vi "CW - Main.vi"() -> ()   [LabVIEW 2017]
doc: "Car Wash Automaion Application VI"
uses:
  Controls/CW - Wash Options.ctl
  Controls/CW - Car Position Control.ctl
  Controls/CW - Car Wash Indicators.ctl
  Controls/CW - Car Wash SM States.ctl
  Controls/CW -  Master Cluster.ctl
panel:
  in  "current time":timestamp
  in  "Stop":bool
  out "Elapsed Time (sec)":dbl format="%#.2g"
  out "Wash Indicators":T1
  in  "Car Position Slider":T2 scale=0.0..4.0
  out "Wash Entry":bool
  in  "Start":bool
  in  "Wash Options":T3
  # "Entry Console"
  # "Car Wash Display"
  # "The wash options controls allow you to determine which cycles will be performed.  \n\nIf none are selected, the High Pressure Wash cycle is the default.  \n\nOnce the start button is clicked, the wash begins."
  # "The Wash Entry LED indicates whether or not the wash in vacant or in use.\n\nThe Wash Indicator LEDs indicate the current status when the wash is in use.\n\nThe Elapsed Time indicator shows the progress for the current cycle, only if it is a timed cycle."
  # "Car Position Simulation"
  # "The Car Position Slider allows you to simulate the position of a vehicle in the wash.\n\nThe vehicle must be at the correct station for the each wash cycle to work.  The cycles that are completed at each station are indicated below the station number.\n\nIf the Vehicle Out of Position LED above is green, adjust your position to the appropraite station."
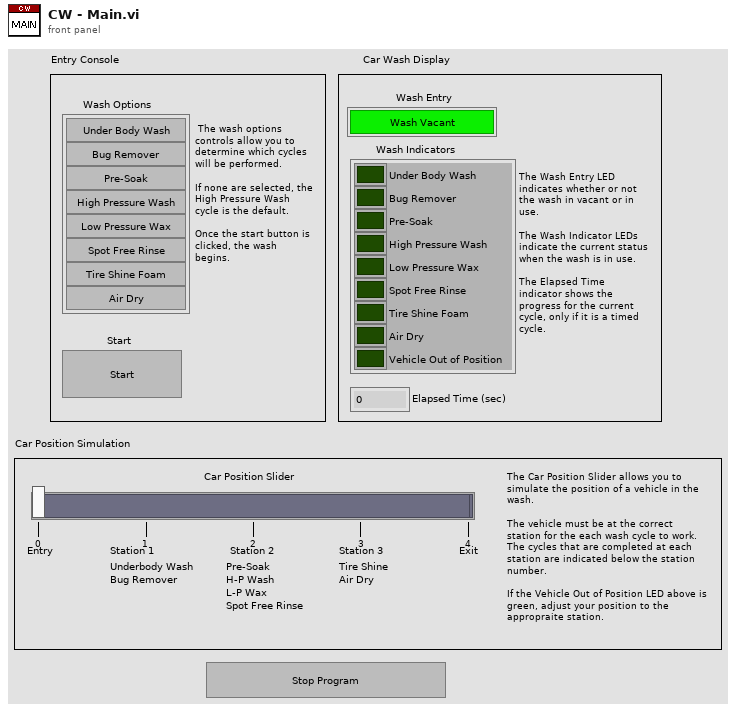
[diagram p1: front panel]
types:
  T1 = typedef "CW - Car Wash Indicators.ctl" = cluster{"Under Body Wash":bool, "Bug Remover":bool, "Pre-Soak":bool, "High Pressure Wash":bool, "Low Pressure Wax":bool, "Spot Free Rinse":bool, "Tire Shine Foam":bool, "Air Dry":bool, "Vehicle Out of Position":bool}
  T2 = typedef "CW - Car Position Control.ctl" = i32
  T3 = typedef "CW - Wash Options.ctl" = cluster{"Under Body Wash":bool, "Bug Remover":bool, "Pre-Soak":bool, "High Pressure Wash":bool, "Low Pressure Wax":bool, "Spot Free Rinse":bool, "Tire Shine Foam":bool, "Air Dry":bool}
  T4 = typedef "CW -  Master Cluster.ctl" = cluster{"Expected_position":i32, "Current_position":i32, "Elapsed Time (sec)":dbl, "Start Timer":bool, "Wash Entry":bool, "Controls Enable":bool, "Time Elapsed":bool, "Wash Step done":bool, "Wash Options":T3, "Wash Indicators":T1}
  T5 = typedef "CW - Car Wash SM States.ctl" = enum16{"Initialize", "Poll", "WaitTime at CW", "Get Data", "Unable/Disable Controls", "Update Indicators", "Start CW", "Entry", "Station 1", "Station 2", "Station 3", "Exit CarWash", "Exit", "Error"}
  T6 = cluster{"Wash Indicators[0]":bool, "Wash Indicators[1]":bool, "Wash Indicators[2]":bool, "Wash Indicators[3]":bool, "Wash Indicators[4]":bool, "Wash Indicators[5]":bool, "Wash Indicators[6]":bool, "Wash Indicators[7]":bool, "Wash Indicators[8]":bool}
  T7 = enum8{"Enabled", "Disabled", "Disabled and Grayed Out"}
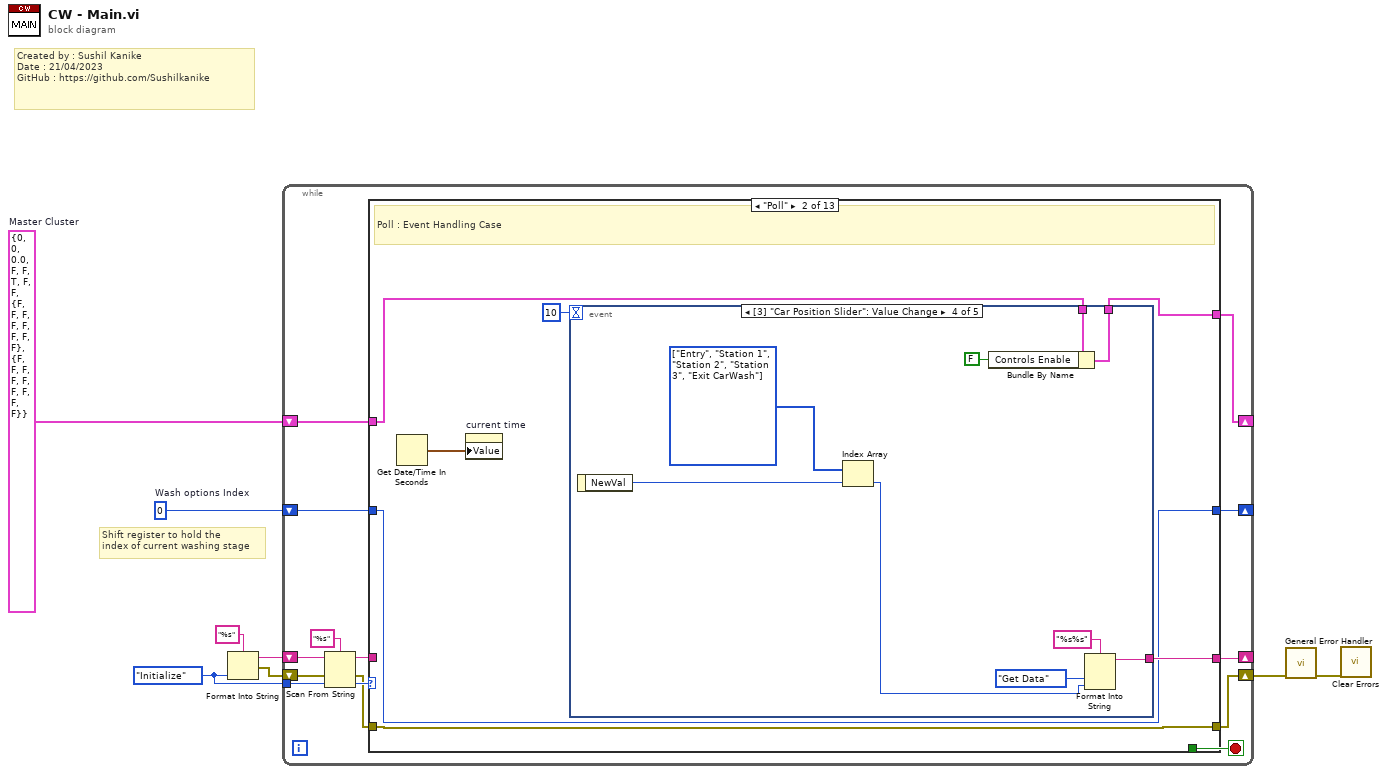
[diagram p0: block diagram]
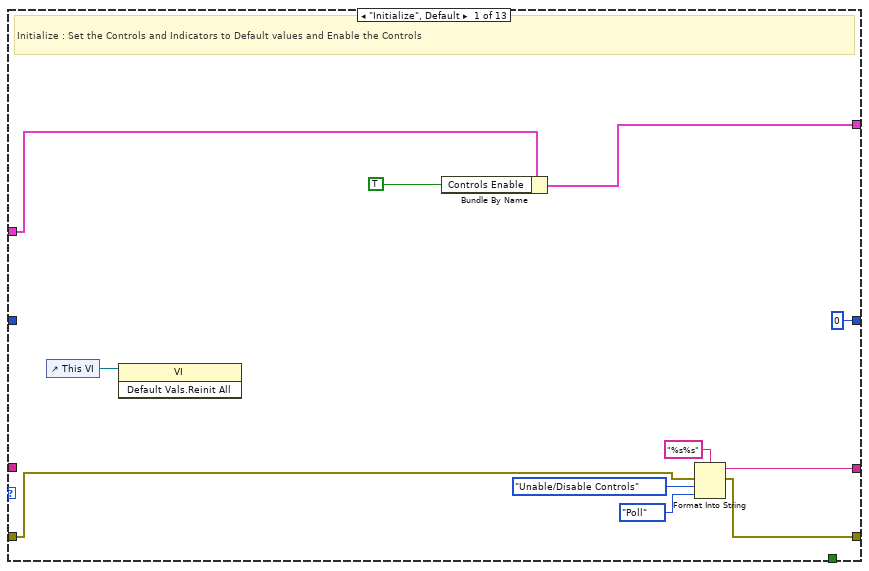
[diagram p2: hidden frame]
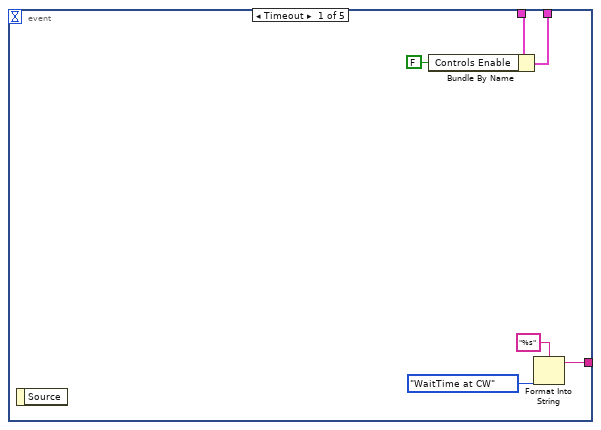
[diagram p3: hidden frame]
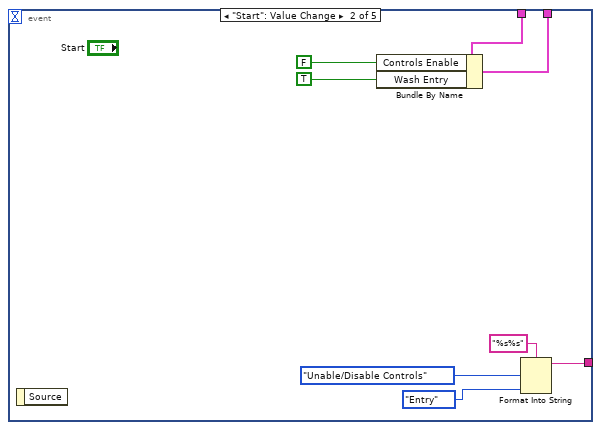
[diagram p4: hidden frame]
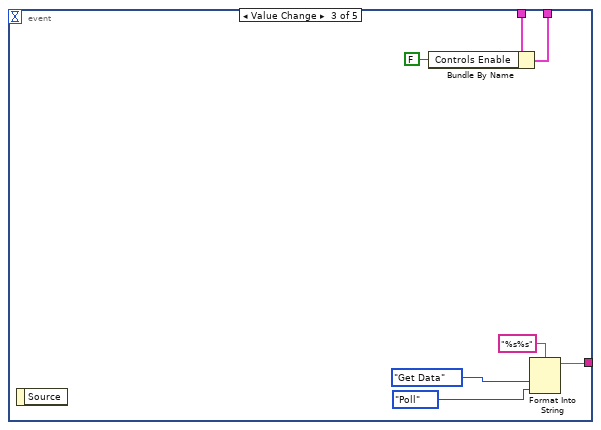
[diagram p5: hidden frame]
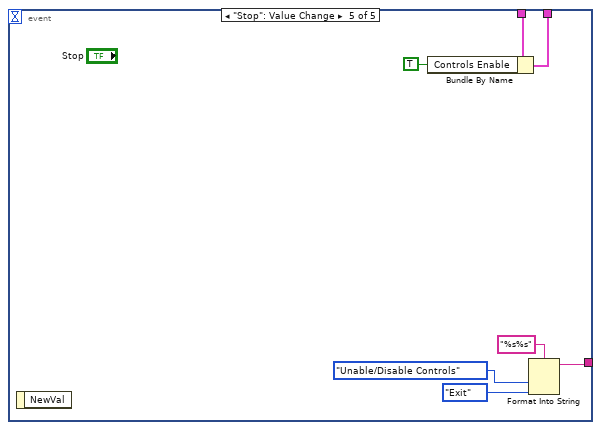
[diagram p6: hidden frame]
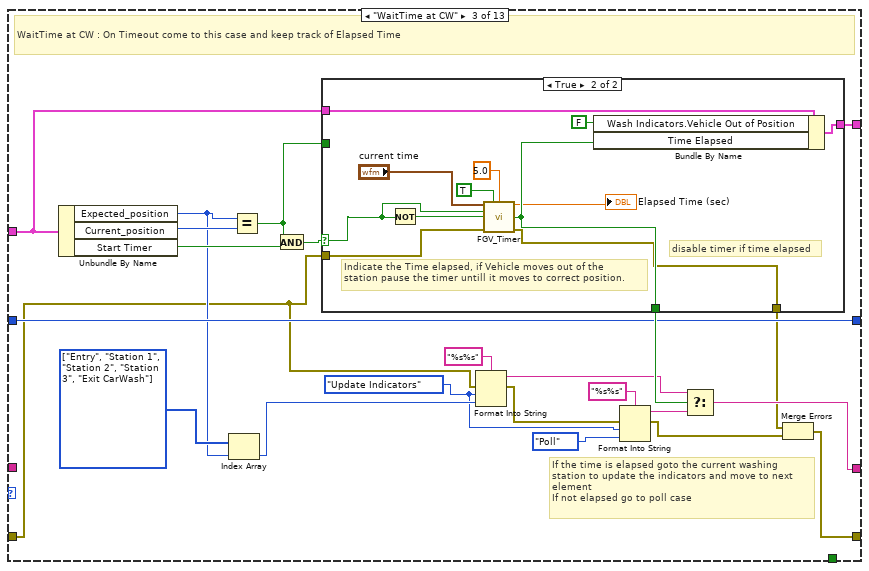
[diagram p7: hidden frame]
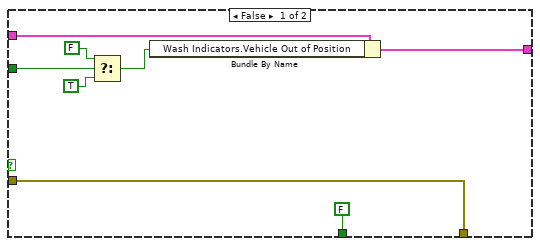
[diagram p8: hidden frame]
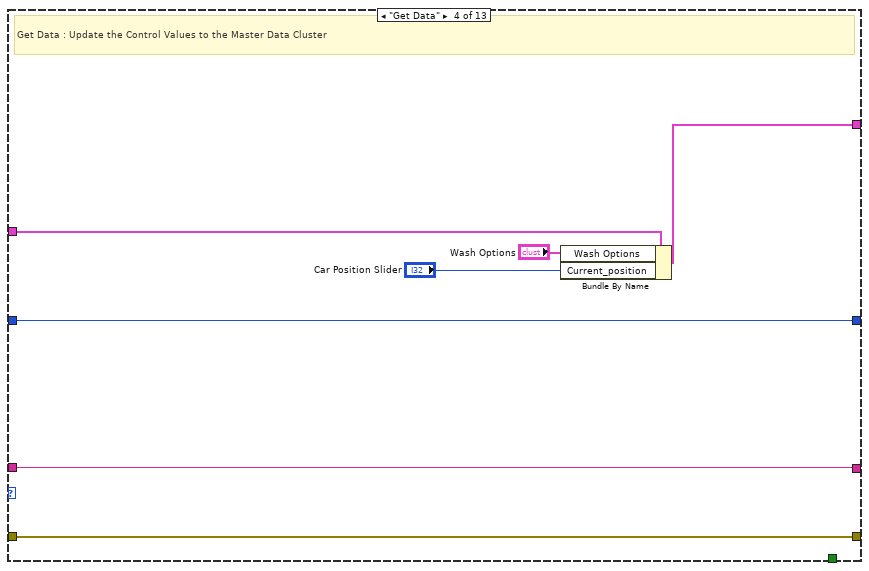
[diagram p9: hidden frame]
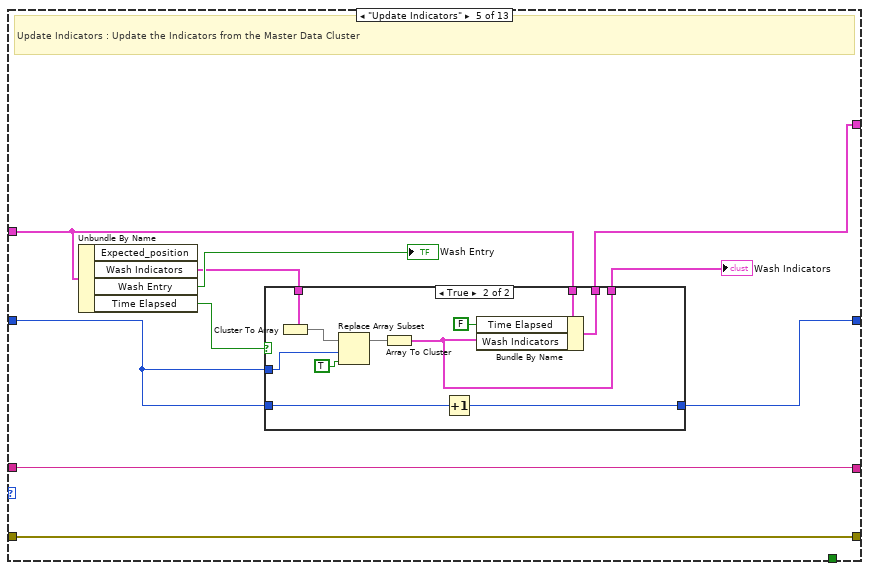
[diagram p10: hidden frame]
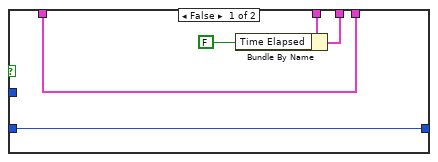
[diagram p11: hidden frame]
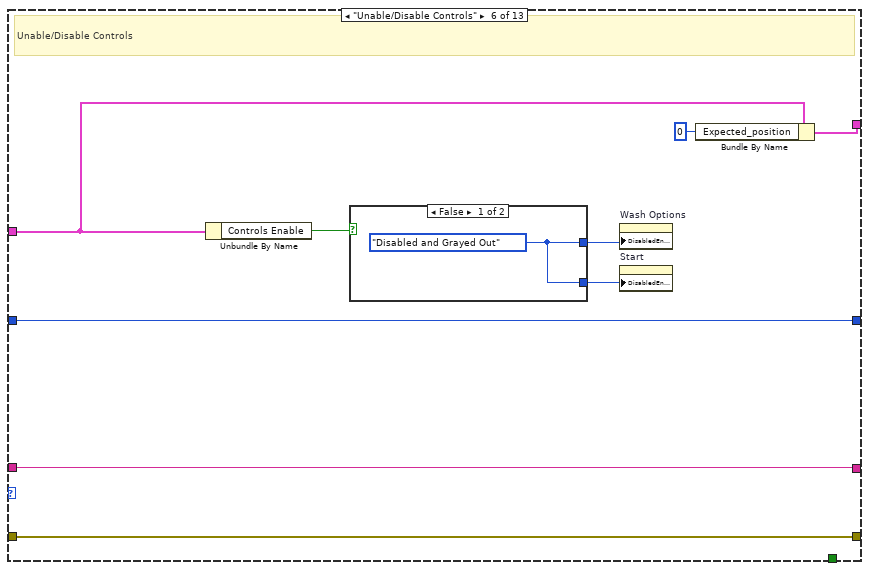
[diagram p12: hidden frame]
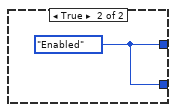
[diagram p13: hidden frame]
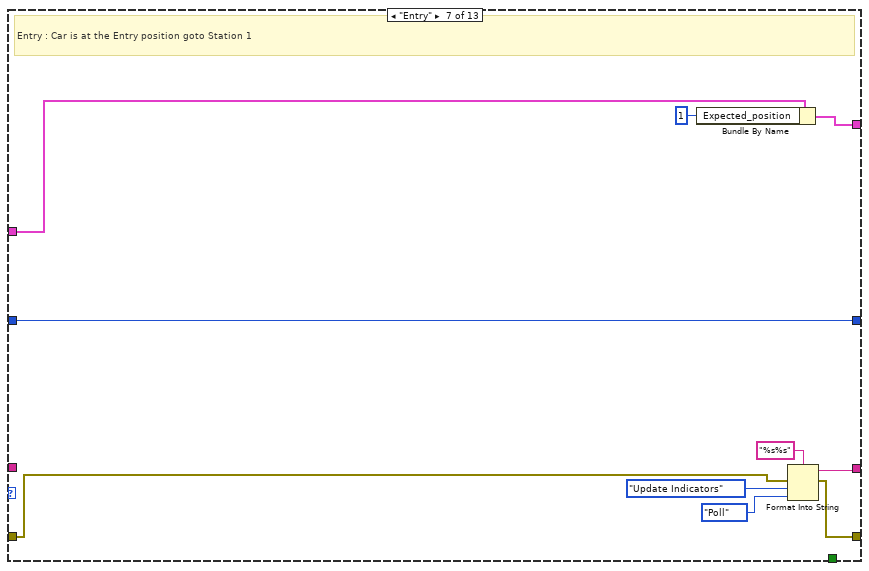
[diagram p14: hidden frame]
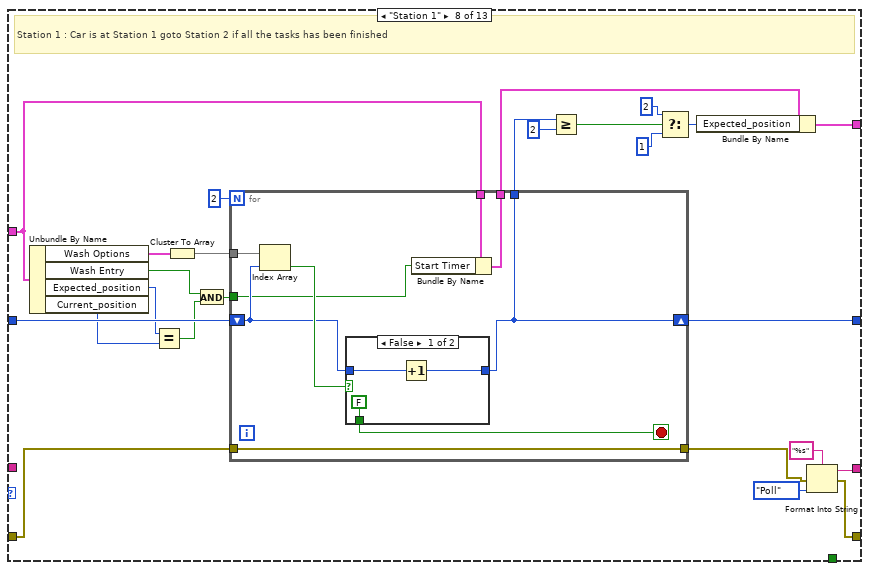
[diagram p15: hidden frame]
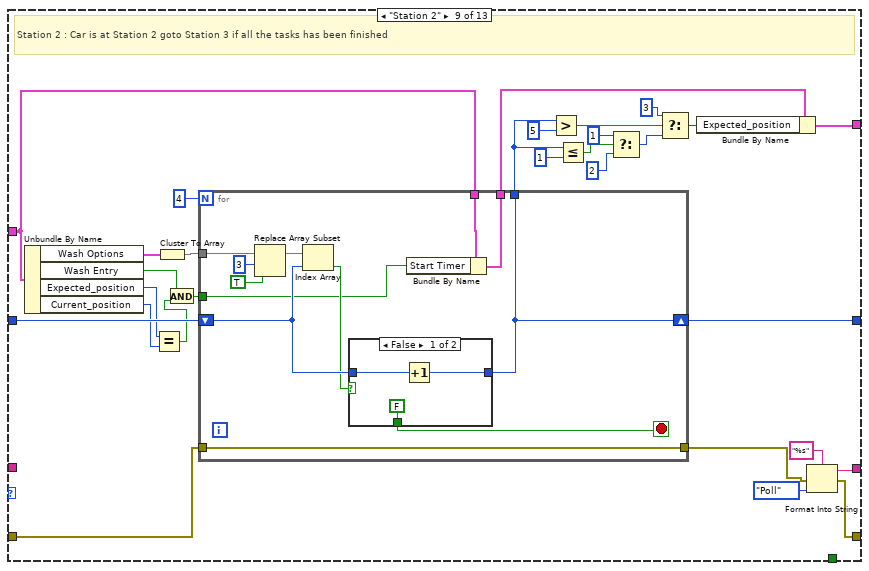
[diagram p17: hidden frame]
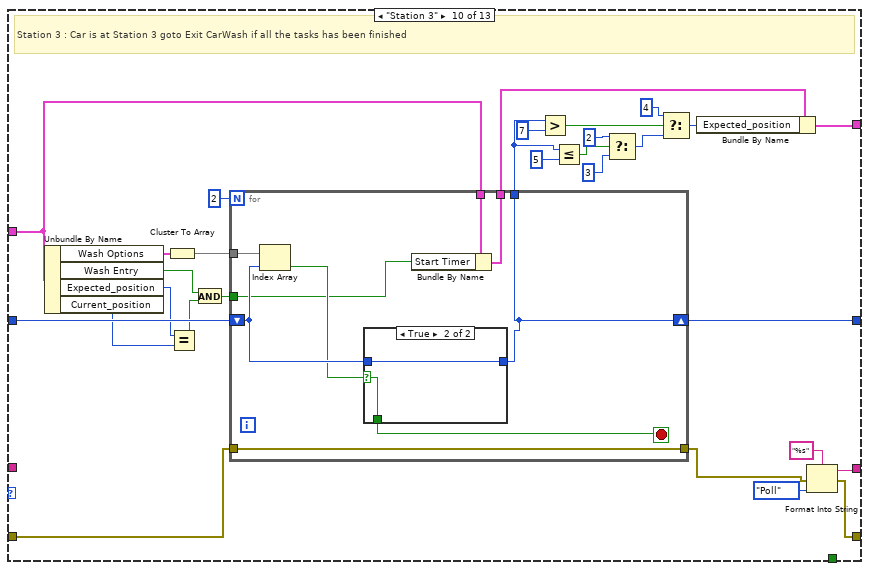
[diagram p19: hidden frame]
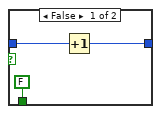
[diagram p20: hidden frame]
diagram:
  w4 = 0  # Wash options Index
  w5 = T4 {"Expected_position"=0, "Current_position"=0, "Elapsed Time (sec)"=0.0, "Start Timer"=FALSE, "Wash Entry"=FALSE, "Controls Enable"=TRUE, "Time Elapsed"=FALSE, "Wash Step done"=FALSE, "Wash Options"={"Under Body Wash"=FALSE, "Bug Remover"=FALSE, "Pre-Soak"=FALSE, "High Pressure Wash"=FALSE, "Low Pressure Wax"=FALSE, "Spot Free Rinse"=FALSE, "Tire Shine Foam"=FALSE, "Air Dry"=FALSE}, "Wash Indicators"={"Under Body Wash"=FALSE, "Bug Remover"=FALSE, "Pre-Soak"=FALSE, "High Pressure Wash"=FALSE, "Low Pressure Wax"=FALSE, "Spot Free Rinse"=FALSE, "Tire Shine Foam"=FALSE, "Air Dry"=FALSE, "Vehicle Out of Position"=FALSE}}  # Master Cluster
  w6 = CW_-_Car_Wash_SM_States."Initialize" ("Car Wash SM States")
  # "Created by : Sushil Kanike\nDate : 21/04/2023 \nGitHub : https://github.com/Sushilkanike"
  # "Shift register to hold the\nindex of current washing stage"
  n1 = Format Into String(format string="%s", w6) -> (resulting string=w7:string, error out=w8:errorcluster)  [unwired: 2 in]
  n2 = while {
    shift-right: [w17] -> _
    shift-left: w7 -> [w16]
    tunnel: w6 -> [w21]
    shift-right: [w14] -> _
    shift-left: w5 -> [w15]
    shift-right: [w13] -> _
    shift-left: w4 -> [w11]
    shift-right: [w9] -> w2
    shift-left: w8 -> [w22]
    stop <- w18 stop-if-true
    n3 = Scan From String(format string="%s", input string=w16, error in=w22, default 1=w21) -> (remaining string=w12:string, error out=w10:errorcluster, output 1=w20:T5)  [unwired: 1 in, 1 out]
    n4 = case shown="\"Poll\"" w20 {
      tunnel: [_ _ _ _ _ _ _ _ _ _ _ TRUE _] -> w18
      tunnel: [w33 w39 w94 w122 w136 w155 w170 w197 w239 w285 w319 w327 w333] -> w17
      tunnel: w15 -> [w28 w37 w93 w127 w129 w159 w173 w193 w222 w281 w324 w329 w335]
      tunnel: [w27 w36 w92 w126 w133 w158 w174 w184 w242 w288 w325 w329 w335] -> w14
      tunnel: w11 -> [_ w38 w89 w123 w131 w156 w169 w192 w234 w279 w305 w328 w334]
      tunnel: [0 w38 w89 w123 w130 w156 w169 w191 w229 w274 w305 w328 w334] -> w13
      tunnel: w12 -> [_ _ _ w122 w136 w155 _ _ _ _ _ w327 w333]
      tunnel: w10 -> [w24 w34 w82 w121 w128 w154 w166 w177 w216 w262 w304 w326 w332]
      tunnel: [w23 w34 w78 w121 w128 w154 w165 w176 w214 w260 w303 w326 w332] -> w9
      frame "Initialize", Default {
        # "Initialize : Set the Controls and Indicators to Default values and Enable the Controls"
        n5 = control-ref of="This VI"() -> (w30:refnum<vi>)
        n6 = invoke class="VI" method="Default Vals.Reinit All"(reference=w30) -> ()  [unwired: 2 in, 3 out]
        n7 = Bundle By Name(cluster=w28, "Controls Enable"=TRUE) -> (w27:T4)
        n8 = Format Into String(format string="%s%s", error in=w24, CW_-_Car_Wash_SM_States."Unable/Disable Controls" ("Car Wash SM States"), CW_-_Car_Wash_SM_States."Poll" ("Car Wash SM States")) -> (resulting string=w33:string, error out=w23:errorcluster)  [unwired: 1 in]
      }
      frame "Poll" {
        # "Poll : Event Handling Case"
        n9 = Get Date/Time In Seconds() -> (seconds since 1Jan1904=w35:timestamp)
        n10 = property on="current time" class="AbsTime (strict)"("Value"=w35) -> ()  [unwired: 2 in, 2 out]
        n11 = event shown="[3] \"Car Position Slider\": Value Change" {
          selector: _ -> [_ _ _ _ _]
          dyn-events: _ -> [_ _ _ _ _]
          timeout: 10 -> [_ _ _ _ _]
          tunnel: [w46 w52 w59 w68 w76] -> w39
          tunnel: w37 -> [w42 w50 w57 w62 w74]
          tunnel: [w41 w49 w56 w63 w73] -> w36
          event Timeout {
            n12 = event-data() -> ()  [unwired: 1 in, 1 out]
            n13 = Bundle By Name(cluster=w42, "Controls Enable"=FALSE) -> (w41:T4)
            n14 = Format Into String(format string="%s", CW_-_Car_Wash_SM_States."WaitTime at CW" ("Car Wash SM States")) -> (resulting string=w46:string)  [unwired: 2 in, 1 out]
          }
          event "Start": Value Change {
            n15 = event-data() -> ()  [unwired: 1 in, 1 out]
            n16 = Bundle By Name(cluster=w50, "Controls Enable"=FALSE, "Wash Entry"=TRUE ("Time Elapsed")) -> (w49:T4)
            n17 = Format Into String(format string="%s%s", CW_-_Car_Wash_SM_States."Unable/Disable Controls" ("Car Wash SM States"), CW_-_Car_Wash_SM_States."Entry" ("Car Wash SM States")) -> (resulting string=w52:string)  [unwired: 2 in, 1 out]
          }
          event Value Change {
            n18 = event-data() -> ()  [unwired: 1 in, 1 out]
            n19 = Bundle By Name(cluster=w57, "Controls Enable"=FALSE) -> (w56:T4)
            n20 = Format Into String(format string="%s%s", CW_-_Car_Wash_SM_States."Get Data" ("Car Wash SM States"), CW_-_Car_Wash_SM_States."Poll" ("Car Wash SM States")) -> (resulting string=w59:string)  [unwired: 2 in, 1 out]
          }
          event Value Change {
            w67 = T5[] [enum."Entry", enum."Station 1", enum."Station 2", enum."Station 3", enum."Exit CarWash"] items=["Initialize", "Poll", "WaitTime at CW", "Get Data", "Unable/Disable Controls", "Update Indicators", "Start CW", "Entry", "Station 1", "Station 2", "Station 3", "Exit CarWash", "Exit", "Error"]
            n21 = event-data() -> ("NewVal"=w66:T2)  [unwired: 1 in]
            n22 = Index Array(array=w67, index=w66) -> (element=w65:T5)
            n23 = Bundle By Name(cluster=w62, "Controls Enable"=FALSE) -> (w63:T4)
            n24 = Format Into String(format string="%s%s", CW_-_Car_Wash_SM_States."Get Data" ("Car Wash SM States"), w65) -> (resulting string=w68:string)  [unwired: 2 in, 1 out]
          }
          event "Stop": Value Change {
            n25 = event-data() -> ()  [unwired: 1 in, 1 out]
            n26 = Bundle By Name(cluster=w74, "Controls Enable"=TRUE) -> (w73:T4)
            n27 = Format Into String(format string="%s%s", CW_-_Car_Wash_SM_States."Unable/Disable Controls" ("Car Wash SM States"), CW_-_Car_Wash_SM_States."Exit" ("Car Wash SM States")) -> (resulting string=w76:string)  [unwired: 2 in, 1 out]
          }
        }
      }
      frame "WaitTime at CW" {
        w84 = CW_-_Car_Wash_SM_States."Update Indicators" ("Car Wash SM States")
        w95 = T5[] [enum."Entry", enum."Station 1", enum."Station 2", enum."Station 3", enum."Exit CarWash"] items=["Initialize", "Poll", "WaitTime at CW", "Get Data", "Unable/Disable Controls", "Update Indicators", "Start CW", "Entry", "Station 1", "Station 2", "Station 3", "Exit CarWash", "Exit", "Error"]
        # "If the time is elapsed goto the current washing \nstation to update the indicators and move to next\nelement\nIf not elapsed go to poll case"
        # "WaitTime at CW : On Timeout come to this case and keep track of Elapsed Time"
        n28 = Unbundle By Name(w93) -> ("Expected_position"=w83:i32, "Current_position"=w86:i32, "Start Timer"=w88:bool)
        n29 = Index Array(array=w95, index=w83) -> (element=w87:T5)
        n30 = Equal?(x=w83, y=w86) -> (x = y?=w90:bool)
        n31 = And(x=w90, y=w88) -> (x .and. y?=w91:bool)
        n32 = case shown="True" w91 {
          selector: w91 -> [_ w114]
          tunnel: [FALSE ("Threshold Trigger") w112] -> w98
          tunnel: w93 -> [w108 w119]
          tunnel: [w107 w118] -> w92
          tunnel: w90 -> [w102 _]
          tunnel: w82 -> [w101 w111]
          tunnel: [w101 w110] -> w80
          frame False {
            n33 = Select(t=FALSE ("Wash Indicators.Vehicle Out of Position"), s=w102, f=TRUE ("Wash Indicators.Vehicle Out of Position")) -> (s? t:f=w104:bool)
            n34 = Bundle By Name(cluster=w108, "Wash Indicators.Vehicle Out of Position"=w104) -> (w107:T4)
          }
          frame True {
            # "disable timer if time elapsed"
            # "Indicate the Time elapsed, if Vehicle moves out of the\nstation pause the timer untill it moves to correct position."
            n35 = Not(x=w114) -> (.not. x?=w115:bool)
            n36 = call "FGV_Timer.vi"("Get Date/Time In Seconds"="current time", "Threshold Set"=TRUE, "Threshold"=5.0, "Start"=w114, "Pause"=w115, "error in"=w111) -> ("Elapsed Time"=→"Elapsed Time (sec)":dbl, "Threshold Trigger"=w112:bool, "error out"=w110:errorcluster)  [unwired: 7 in]
            n37 = Bundle By Name(cluster=w119, "Wash Indicators.Vehicle Out of Position"=FALSE, "Time Elapsed"=w112) -> (w118:T4)
          }
        }
        n38 = Format Into String(format string="%s%s", error in=w82, w84, w87) -> (resulting string=w96:string, error out=w81:errorcluster)  [unwired: 1 in]
        n39 = Format Into String(format string="%s%s", error in=w81, w84, CW_-_Car_Wash_SM_States."Poll" ("Car Wash SM States")) -> (resulting string=w99:string, error out=w79:errorcluster)  [unwired: 1 in]
        n40 = Select(t=w96, s=w98, f=w99) -> (s? t:f=w94:string)
        n41 = Merge Errors(w80, w79) -> (w78:errorcluster)
      }
      frame "Get Data" {
        # "Get Data : Update the Control Values to the Master Data Cluster"
        n42 = Bundle By Name(cluster=w127, "Wash Options"="Wash Options", "Current_position"="Car Position Slider") -> (w126:T4)
      }
      frame "Update Indicators" {
        # "Update Indicators : Update the Indicators from the Master Data Cluster"
        n43 = Unbundle By Name(w129) -> ("Wash Indicators"=w134:T1, "Wash Entry"=→"Wash Entry":bool, "Time Elapsed"=w135:bool)  [unwired: 1 out]
        n44 = case shown="True" w135 {
          tunnel: w134 -> [w139 w150]
          tunnel: w131 -> [_ w144]
          tunnel: w129 -> [w141 w149]
          tunnel: [w140 w148] -> w133
          tunnel: [w139 w146] -> w132
          tunnel: w131 -> [w138 w145]
          tunnel: [w138 w143] -> w130
          frame False {
            n45 = Bundle By Name(cluster=w141, "Time Elapsed"=FALSE) -> (w140:T4)
          }
          frame True {
            n46 = Cluster To Array(cluster=w150) -> (array=w152:bool[])
            n47 = Replace Array Subset(array=w152, new element=TRUE ("new element/subarray"), index=w144) -> (w153:bool[])
            n48 = Array To Cluster(array=w153) -> (cluster=w146:T6)
            n49 = Increment(x=w145) -> (x+1=w143:i32)
            n50 = Bundle By Name(cluster=w149, "Time Elapsed"=FALSE, "Wash Indicators"=w146) -> (w148:T4)
          }
        }
        "Wash Indicators" <- w132
      }
      frame "Unable/Disable Controls" {
        # "Unable/Disable Controls"
        n51 = Unbundle By Name(w159) -> ("Controls Enable"=w160:bool)
        n52 = case shown="False" w160 {
          tunnel: [w163 w164] -> w162
          tunnel: [w163 w164] -> w161
          frame False {
            w163 = T7."Disabled and Grayed Out" ("Disabled")
          }
          frame True {
            w164 = T7."Enabled" ("Disabled")
          }
        }
        n53 = property on="Wash Options" class="Clust (strict)"("DisabledEnum"=w162) -> ()  [unwired: 2 in, 2 out]
        n54 = property on="Start" class="Bool"("DisabledEnum"=w161) -> ()  [unwired: 2 in, 2 out]
        n55 = Bundle By Name(cluster=w159, "Expected_position"=0) -> (w158:T4)
      }
      frame "Entry" {
        # "Entry : Car is at the Entry position goto Station 1"
        n56 = Bundle By Name(cluster=w173, "Expected_position"=1) -> (w174:T4)
        n57 = Format Into String(format string="%s%s", error in=w166, CW_-_Car_Wash_SM_States."Update Indicators" ("Car Wash SM States"), CW_-_Car_Wash_SM_States."Poll" ("Car Wash SM States")) -> (resulting string=w170:string, error out=w165:errorcluster)  [unwired: 1 in]
      }
      frame "Station 1" {
        # "Station 1 : Car is at Station 1 goto Station 2 if all the tasks has been finished"
        n58 = Unbundle By Name(w193) -> ("Wash Options"=w196:T3, "Wash Entry"=w179:bool, "Expected_position"=w182:i32, "Current_position"=w181:i32)
        n59 = Equal?(x=w182, y=w181) -> (x = y?=w178:bool)
        n60 = Cluster To Array(cluster=w196) -> (array=w195:bool[])
        n61 = And(x=w179, y=w178) -> (x .and. y?=w180:bool)
        n62 = for {
          N: 2 -> [_]
          tunnel: w195 -> [w208]
          tunnel: w193 -> [w207]
          tunnel: [w206] -> w186
          tunnel: [w202] -> w185
          tunnel: w180 -> [w201]
          shift-right: [w202] -> w191
          shift-left: w192 -> [w203]
          tunnel: w177 -> [w200]
          tunnel: [w200] -> w175
          stop <- w204 stop-if-true
          n63 = Index Array(array=w208, index=w203) -> (element=w205:bool)
          n64 = case shown="False" w205 {
            selector: w205 -> [_ w213]
            tunnel: [FALSE w213] -> w204
            tunnel: w203 -> [w210 w212]
            tunnel: [w209 w212] -> w202
            frame False {
              n65 = Increment(x=w210) -> (x+1=w209:i32)
            }
            frame True {
            }
          }
          n66 = Bundle By Name(cluster=w207, "Start Timer"=w201) -> (w206:T4)
        }
        n67 = Greater Or Equal?(x=w185, y=2) -> (x >= y?=w190:bool)
        n68 = Select(t=2 ("Expected_position"), s=w190, f=1) -> (s? t:f=w187:i32)
        n69 = Bundle By Name(cluster=w186, "Expected_position"=w187) -> (w184:T4)
        n70 = Format Into String(format string="%s", error in=w175, CW_-_Car_Wash_SM_States."Poll" ("Car Wash SM States")) -> (resulting string=w197:string, error out=w176:errorcluster)  [unwired: 1 in]
      }
      frame "Station 2" {
        # "Station 2 : Car is at Station 2 goto Station 3 if all the tasks has been finished"
        n71 = Unbundle By Name(w222) -> ("Wash Options"=w238:T3, "Wash Entry"=w218:bool, "Expected_position"=w221:i32, "Current_position"=w220:i32)
        n72 = Equal?(x=w221, y=w220) -> (x = y?=w219:bool)
        n73 = Cluster To Array(cluster=w238) -> (array=w237:bool[])
        n74 = And(x=w218, y=w219) -> (x .and. y?=w217:bool)
        n75 = for {
          N: 4 -> [_]
          tunnel: w237 -> [w247]
          tunnel: w222 -> [w254]
          tunnel: [w253] -> w235
          tunnel: [w251] -> w225
          tunnel: w217 -> [w248]
          shift-right: [w251] -> w229
          shift-left: w234 -> [w252]
          tunnel: w216 -> [w243]
          tunnel: [w243] -> w215
          stop <- w249 stop-if-true
          n76 = Replace Array Subset(array=w247, new element=TRUE ("new element/subarray"), index=3) -> (w246:bool[])
          n77 = Index Array(array=w246, index=w252) -> (element=w250:bool)
          n78 = case shown="False" w250 {
            selector: w250 -> [_ w259]
            tunnel: [FALSE w259] -> w249
            tunnel: w252 -> [w256 w258]
            tunnel: [w255 w258] -> w251
            frame False {
              n79 = Increment(x=w256) -> (x+1=w255:i32)
            }
            frame True {
            }
          }
          n80 = Bundle By Name(cluster=w254, "Start Timer"=w248) -> (w253:T4)
        }
        n81 = Greater?(x=w225, y=5) -> (0:w233:bool)
        n82 = Less Or Equal?(x=w225, y=1) -> (x <= y?=w227:bool)
        n83 = Select(t=1, s=w227, f=2 ("Expected_position")) -> (s? t:f=w223:i32)
        n84 = Select(t=3 ("Expected_position"), s=w233, f=w223) -> (s? t:f=w230:i32)
        n85 = Bundle By Name(cluster=w235, "Expected_position"=w230) -> (w242:T4)
        n86 = Format Into String(format string="%s", error in=w215, CW_-_Car_Wash_SM_States."Poll" ("Car Wash SM States")) -> (resulting string=w239:string, error out=w214:errorcluster)  [unwired: 1 in]
      }
      frame "Station 3" {
        # "Station 3 : Car is at Station 3 goto Exit CarWash if all the tasks has been finished"
        n87 = Unbundle By Name(w281) -> ("Wash Options"=w284:T3, "Wash Entry"=w264:bool, "Expected_position"=w267:i32, "Current_position"=w266:i32)
        n88 = Cluster To Array(cluster=w284) -> (array=w283:bool[])
        n89 = Equal?(x=w267, y=w266) -> (x = y?=w263:bool)
        n90 = And(x=w264, y=w263) -> (x .and. y?=w265:bool)
        n91 = for {
          N: 2 -> [_]
          tunnel: w283 -> [w297]
          tunnel: w281 -> [w296]
          tunnel: [w295] -> w280
          tunnel: [w293] -> w269
          tunnel: w265 -> [w290]
          shift-right: [w293] -> w274
          shift-left: w279 -> [w294]
          tunnel: w262 -> [w289]
          tunnel: [w289] -> w261
          stop <- w292 stop-if-true
          n92 = Index Array(array=w297, index=w294) -> (element=w291:bool)
          n93 = case shown="True" w291 {
            selector: w291 -> [_ w302]
            tunnel: [FALSE w302] -> w292
            tunnel: w294 -> [w299 w301]
            tunnel: [w298 w301] -> w293
            frame False {
              n94 = Increment(x=w299) -> (x+1=w298:i32)
            }
            frame True {
            }
          }
          n95 = Bundle By Name(cluster=w296, "Start Timer"=w290) -> (w295:T4)
        }
        n96 = Greater?(x=w269, y=7) -> (0:w278:bool)
        n97 = Less Or Equal?(x=w269, y=5) -> (x <= y?=w272:bool)
        n98 = Select(t=2, s=w272, f=3 ("Expected_position")) -> (s? t:f=w270:i32)
        n99 = Select(t=4 ("Expected_position"), s=w278, f=w270) -> (s? t:f=w275:i32)
        n100 = Bundle By Name(cluster=w280, "Expected_position"=w275) -> (w288:T4)
        n101 = Format Into String(format string="%s", error in=w261, CW_-_Car_Wash_SM_States."Poll" ("Car Wash SM States")) -> (resulting string=w285:string, error out=w260:errorcluster)  [unwired: 1 in]
      }
      frame "Exit CarWash" {
        # "Exit CarWash : Car is at ExitCarWash goto Entry if all the tasks has been finished"
        n102 = Less Or Equal?(x=w305, y=7) -> (x <= y?=w311:bool)
        n103 = Select(t=3 ("y"), s=w311, f=0) -> (s? t:f=w308:i32)
        n104 = Less?(x=w305, y=5) -> (x < y?=w313:bool)
        n105 = Less?(x=w305, y=1) -> (x < y?=w318:bool)
        n106 = Select(t=2 ("y"), s=w313, f=w308) -> (s? t:f=w312:i32)
        n107 = Select(t=1 ("y"), s=w318, f=w312) -> (s? t:f=w306:i32)
        n108 = Bundle By Name(cluster=w324, "Expected_position"=w306, "Controls Enable"=TRUE, "Wash Entry"=TRUE) -> (w325:T4)
        n109 = Format Into String(format string="%s", error in=w304, CW_-_Car_Wash_SM_States."Poll" ("Car Wash SM States")) -> (resulting string=w319:string, error out=w303:errorcluster)  [unwired: 1 in]
      }
      frame "Exit" {
        # "Exit : Set all te Controls to default and Exit the Application"
        n110 = control-ref of="This VI"() -> (w330:refnum<vi>)
        n111 = invoke class="VI" method="Default Vals.Reinit All"(reference=w330) -> ()  [unwired: 2 in, 3 out]
      }
      frame "Error" {
      }
    }
  }
  n112 = call <vilib>:"General Error Handler.vi"("error in (no error)"=w2) -> ("error out"=w1:errorcluster)  [unwired: 10 in, 4 out]
  n113 = call <vilib>:"Clear Errors.vi"("error in (no error)"=w1) -> ()  [unwired: 5 in, 2 out]
